vi "Diagnostics - Workspace Object.vi"() -> ()   [LabVIEW 2019, in "Diagnostics Workspace Object.lvlib"]
doc: "Sample numeric display item."
uses:
  Diagnostics Workspace Object.lvlib
  <vilib>/NI VeriStand/Display Template Support/DisplayTemplateSupport.llb/enum_Display Template Handler Minimal To Widget Msg.ctl
  <vilib>/NI VeriStand/Display Template Support/DisplayTemplateSupport.llb/enum_Display Template Handler Minimal To Workspace.ctl
  Workspace Shared/Types/Workspace.State.ctl
  Workspace Shared/Diagnostics Workspace Shared.lvlib
  <vilib>/NI VeriStand/Execution/Workspace/SystemStateRegEventRef.ctl
  <vilib>/NI VeriStand/Execution/Workspace/NI_VS Workspace ExecutionAPI.lvlib
  <vilib>/NI VeriStand/Execution/Workspace/WorkspaceAPI.ctl
  <vilib>/NI VeriStand/Execution/Workspace/SystemStateEventRef.ctl
  Workspace Shared/Types/UI.Refs.ctl
  <vilib>/NI VeriStand/Execution/Workspace/Target State.ctl
  <vilib>/NI VeriStand/Execution/Workspace/Target State Info.ctl
  Workspace Shared/Types/Workspace.SavedState.ctl
  Addon/Addon Shared/Types/Protocol.ctl
  Addon/Addon Shared/Diagnostics Addon Shared.lvlib
  <vilib>/NI VeriStand/Display Template Support/DisplayTemplateSupport.llb/sub_Display Template Handler Custom.vi
  NationalInstruments.VeriStand.ClientAPI
  NationalInstruments.VeriStand.SystemStorage
  Addon/Addon Shared/Types/Command.New.ctl
  APIs/Host Automation API/Diagnostics Host Automation API.lvlib
  Addon/Addon Shared/Types/DTC.Descriptor.Override.ctl
  Addon/Addon Shared/Types/Command.ReadDTC.ctl
  <vilib>/NI VeriStand/Execution/Workspace/NI VeriStand - Set Single Channel Value.vi
  <vilib>/NI VeriStand/Execution/Workspace/NI VeriStand - Get Multiple Channel Values.vi
  <vilib>/xnet/xnet.llb/XNET Frame Type CAN.ctl
  <vilib>/xnet/xnet.llb/XNET Frame CAN.ctl
  SubModules/CAN-Streaming-Support/UIs/Workspace Shared/Types/Host Stream Queue Command.ctl
  SubModules/CAN-Streaming-Support/UIs/Workspace Shared/CAN Stream Support Workspace Shared.lvlib
  SubModules/CAN-Streaming-Support/UIs/Workspace Shared/Types/Host Stream Queue Type.ctl
  SubModules/CAN-Streaming-Support/UIs/Workspace Shared/Types/Host Stream Queue Refs.ctl
  <vilib>/NI VeriStand/Display Template Support/DisplayTemplateSupport.llb/cluster_Screen Item Settings.ctl
  <vilib>/NI VeriStand/Display Template Support/DisplayTemplateSupport.llb/cluster_Graph Scale Settings.ctl
  <vilib>/NI VeriStand/Display Template Support/DisplayTemplateSupport.llb/cluster_Graph Plot Settings.ctl
panel:
  in  "Tab Control":enum32{"Cmd", "Raw", "Read DTCs"}(tab)
  out "Time Stamp":timestamp
  out "CAN Connected?":bool
  in  "Send":bool
  out "VeriStand Error":i64 format="%.0x"
  out "Success?":bool
  in  "Cmd":T1
  in  "Clear":bool
  out "Raw VeriStand Error":errorcluster
  out "Raw Error Byte":u8 format="%.0x"
  in  "Response Required?":bool
  in  "Send Raw":bool
  out "Raw Resp":u8[](array[numeric]) format="%.0x"
  in  "Raw Cmd":u8[](array[numeric]) format="%.0x"
  in  "DTC":u32
  in  "Status":u32
  in  "Failure":u32
  in  "Override Byte Lengths":bool
  in  "Extension":u32 format="%.0x"
  in  "Mask":u32 format="%.0x"
  in  "Mode":u32 format="%.0x"
  in  "Hex":bool=TRUE
  in  "DTCs":string(tree)
  in  "Read DTCs":bool
  out "Device":string
  in  "NIVS.System Definition Root":refnum<k24>
  in  "NIVS.Gateway IP Address":string
  in  "Item.Data":T2
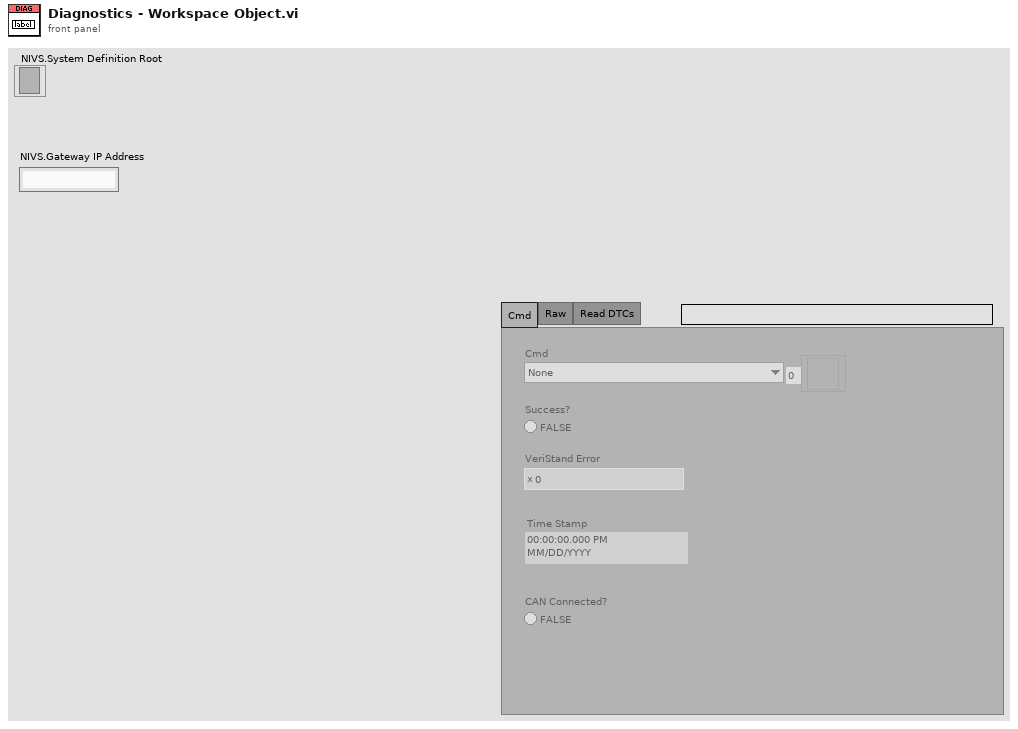
[diagram p1: front panel]
types:
  T1 = typedef "Diagnostics Addon Shared.lvlib/Command.New.ctl" = enum8{"None", "Clear Status Channels", "Read All DIDs", "Read All PIDs", "Configure and Start DPIDs", "Stop DPIDs"}
  T2 = typedef "cluster_Screen Item Settings.ctl" = cluster{"Template VI":string, "Position X":i32, "Position Y":i32, "Custom":string, "Show Title Bar":bool, "ID":i32, "Always On Top":bool, "Allow Resize":bool, "Allow Minimize":bool, "Allow Close":bool, "Size to Screen":bool, "Screen.ID":i32, "State":enum16{"Normal", "New"}, "Title":string, "Window Bounds":cluster{"[0]":i16, "[1]":i16, "[2]":i16, "[3]":i16}, "Channel Ref":u64, "Unit":string, "Default Units?":bool, "Flash Limit?":bool, "Color 1":u32, "Color 2":u32, "Color 3":u32, "Color 4":u32, "Bck Color":u32, "Fore Color":u32, "Limit 1":dbl, "Limit 2":dbl, "Limit 3":dbl, "Limit 4":dbl, "Limit Mode 1":i32, "Limit Mode 2":i32, "Limit Mode 3":i32, "Limit Mode 4":i32, "Scale Precision":i32, "Scale Min":dbl, "Scale Max":dbl, "Format":i32, "Precision":i32, "Background Type":i32, "IDs":i32[], "Units":string[], "Labels":string[], "Scale Factor":dbl, "Scale Offset":dbl, "YScale Index":u32[], "XScale":T3, "YScales":T3[], "Plots":T4[], "Update Period":dbl, "History Length":dbl, "My.Ref":refnum<vi>, "Is Control?":bool, "Channel Paths":string[], "Custom Data":variant}
  T3 = typedef "cluster_Graph Scale Settings.ctl" = cluster{"Format":u8, "Precision":u8, "Fit":u8, "Label":string, "Use Default Label":bool, "Label Visible":bool, "Min":dbl, "Max":dbl}
  T4 = typedef "cluster_Graph Plot Settings.ctl" = cluster{"Bar Style":u8, "Fill To":i16, "Fill/PtColor":u32, "Line Style":u8, "Line Width":u8, "Color":u32, "Interp":u8, "Point Style":u8}
  T5 = typedef "Diagnostics Workspace Shared.lvlib/Workspace.State.ctl" = cluster{"UI.Refs":T6, "Data.PreviousValues":dbl[], "Data.Read":string[], "CachedData.UserEvent":refnum<user-event>, "CachedData":T7, "Addon.Connected?":bool, "NIVS.SysDef":path, "NIVS.SysDefRoot":refnum<k24>, "NIVS.Workspace":T8, "NIVS.UserEventRefs":cluster{"Event Registration Refnum":refnum<event-registration>, "SystemChangeEventRef":T9, "NIVS.Workspace Event":refnum<event-registration>}, "NIVS.SystemStateRefs":T10, "NIVS.LaunchRef":refnum<user-event>, "Data.PendingChange?":bool, "Command.Channel":string, "Diagnostic Protocol":T11, "Channels.Found":bool, "Command.Connect":string, "Mode.Tool?":bool, "Stream.Qs":T12}
  T6 = typedef "Diagnostics Workspace Shared.lvlib/UI.Refs.ctl" = cluster{"Cmd":refnum<vi>, "Success?":refnum<vi>, "VeriStandError":refnum<vi>, "CAN Connected?":refnum<vi>, "DTC":refnum<vi>, "Status":refnum<vi>, "Failure":refnum<vi>, "Override Byte Lengths":refnum<vi>, "Response Required?":refnum<vi>, "Send":refnum<vi>, "Clear":refnum<vi>, "Send Raw":refnum<vi>, "Read DTCs":refnum<vi>, "Raw Cmd":refnum<vi>, "Extension":refnum<vi>, "Mode":refnum<vi>, "Mask":refnum<vi>, "Hex":refnum<vi>, "Raw Resp":refnum<vi>, "Raw Error Byte":refnum<vi>, "Raw VeriStand Error":refnum<vi>, "DTCs":refnum<vi>, "Time Stamp":refnum<vi>, "Device":refnum<vi>, "Pause":refnum<vi>, "Table Control":refnum<vi>, "Sort By ID":refnum<vi>, "Streaming Connected":refnum<vi>, "Enable Stream":refnum<vi>, "CAN State":refnum<vi>, "Direction Filter":refnum<vi>, "Type Filter":refnum<vi>, "Clear History":refnum<vi>, "Filter IDs":refnum<vi>, "Filter Location":refnum<vi>, "Reset Filter":refnum<vi>, "Log":refnum<vi>}
  T7 = typedef "Diagnostics Workspace Shared.lvlib/Workspace.SavedState.ctl" = cluster{"CD Path":string, "CD IP":string}
  T8 = typedef "NI_VS Workspace ExecutionAPI.lvlib/WorkspaceAPI.ctl" = refnum<k24>
  T9 = typedef "NI_VS Workspace ExecutionAPI.lvlib/SystemStateRegEventRef.ctl" = refnum<event-registration>
  T10 = typedef "NI_VS Workspace ExecutionAPI.lvlib/SystemStateEventRef.ctl" = cluster{"CustDatRef":refnum<user-event>, "EvtRef":refnum<k27>, "Target State User Event":refnum<user-event>}
  T11 = typedef "Diagnostics Addon Shared.lvlib/Protocol.ctl" = enum16{"GMLAN", "KWP-2000", "UDS", "User-Defined"}
  T12 = typedef "CAN Stream Support Workspace Shared.lvlib/Host Stream Queue Refs.ctl" = cluster{"Cmd Q":refnum<queue>, "XNET Frames":refnum<queue>}
  T13 = typedef "enum_Display Template Handler Minimal To Workspace.ctl" = cluster{"Operation":enum16{"SetCustomData", "DeleteItem"}, "Data":variant}
  T14 = typedef "enum_Display Template Handler Minimal To Widget Msg.ctl" = enum16{"Stop", "LaunchConfigDialog"}
  T15 = typedef "Diagnostics Addon Shared.lvlib/Command.ReadDTC.ctl" = cluster{"Extension":u32, "Mask":u32, "Mode/Status":u32, "Byte Lengths":T16}
  T16 = typedef "Diagnostics Addon Shared.lvlib/DTC.Descriptor.Override.ctl" = cluster{"Override":bool, "DTC":u32, "Status":u32, "Failure":u32}
  T17 = cluster{"Event Registration Refnum":refnum<event-registration>, "SystemChangeEventRef":T9, "NIVS.Workspace Event":refnum<event-registration>}
  T18 = typedef "Diagnostics Addon Shared.lvlib/UI.Refs.ctl" = cluster{"Cmd":refnum<vi>, "Success?":refnum<vi>, "VeriStandError":refnum<vi>, "CAN Connected?":refnum<vi>, "DTC":refnum<vi>, "Status":refnum<vi>, "Failure":refnum<vi>, "Override Byte Lengths":refnum<vi>, "Response Required?":refnum<vi>, "Send":refnum<vi>, "Clear":refnum<vi>, "Send Raw":refnum<vi>, "Read DTCs":refnum<vi>, "Raw Cmd":refnum<vi>, "Extension":refnum<vi>, "Mode":refnum<vi>, "Mask":refnum<vi>, "Hex":refnum<vi>, "Raw Resp":refnum<vi>, "Raw Error Byte":refnum<vi>, "Raw VeriStand Error":refnum<vi>, "DTCs":refnum<vi>, "Time Stamp":refnum<vi>, "Device":refnum<vi>, "Pause":refnum<vi>, "Table Control":refnum<vi>, "Sort By ID":refnum<vi>, "Streaming Connected":refnum<vi>, "Enable Stream":refnum<vi>, "CAN State":refnum<vi>, "Direction Filter":refnum<vi>, "Type Filter":refnum<vi>, "Clear History":refnum<vi>, "Filter IDs":refnum<vi>, "Filter Location":refnum<vi>, "Reset Filter":refnum<vi>, "Log":refnum<vi>}
  T19 = typedef "Diagnostics Addon Shared.lvlib/HostAutomation.Ref.ctl" = cluster{"TCP Comm":T20, "DTCs":T22}
  T20 = typedef "NI STM.lvlib/TCP Connection Info.ctl" = cluster{"connection ID":refnum<k5>, "meta data":T21[]}
  T21 = typedef "NI STM.lvlib/MetaDataElement.ctl" = string
  T22 = typedef "Diagnostics Addon Shared.lvlib/DTC.Codes.ctl" = cluster{"Value.Code":dbl[], "Value.String":string[], "Value.J2012String":string[], "Status.Code":dbl[], "Status.String":string[]}
  T23 = cluster{"resp":u8[], "error code":u8, "error out":errorcluster}
  T24 = typedef "Diagnostics Addon Shared.lvlib/Command.ReadDTC.DTCs.ctl" = cluster{"Timestamp":dbl, "DTC":dbl, "J2012 String":string, "DTC String":string, "Status":dbl, "Status String":string, "Add Data":dbl}
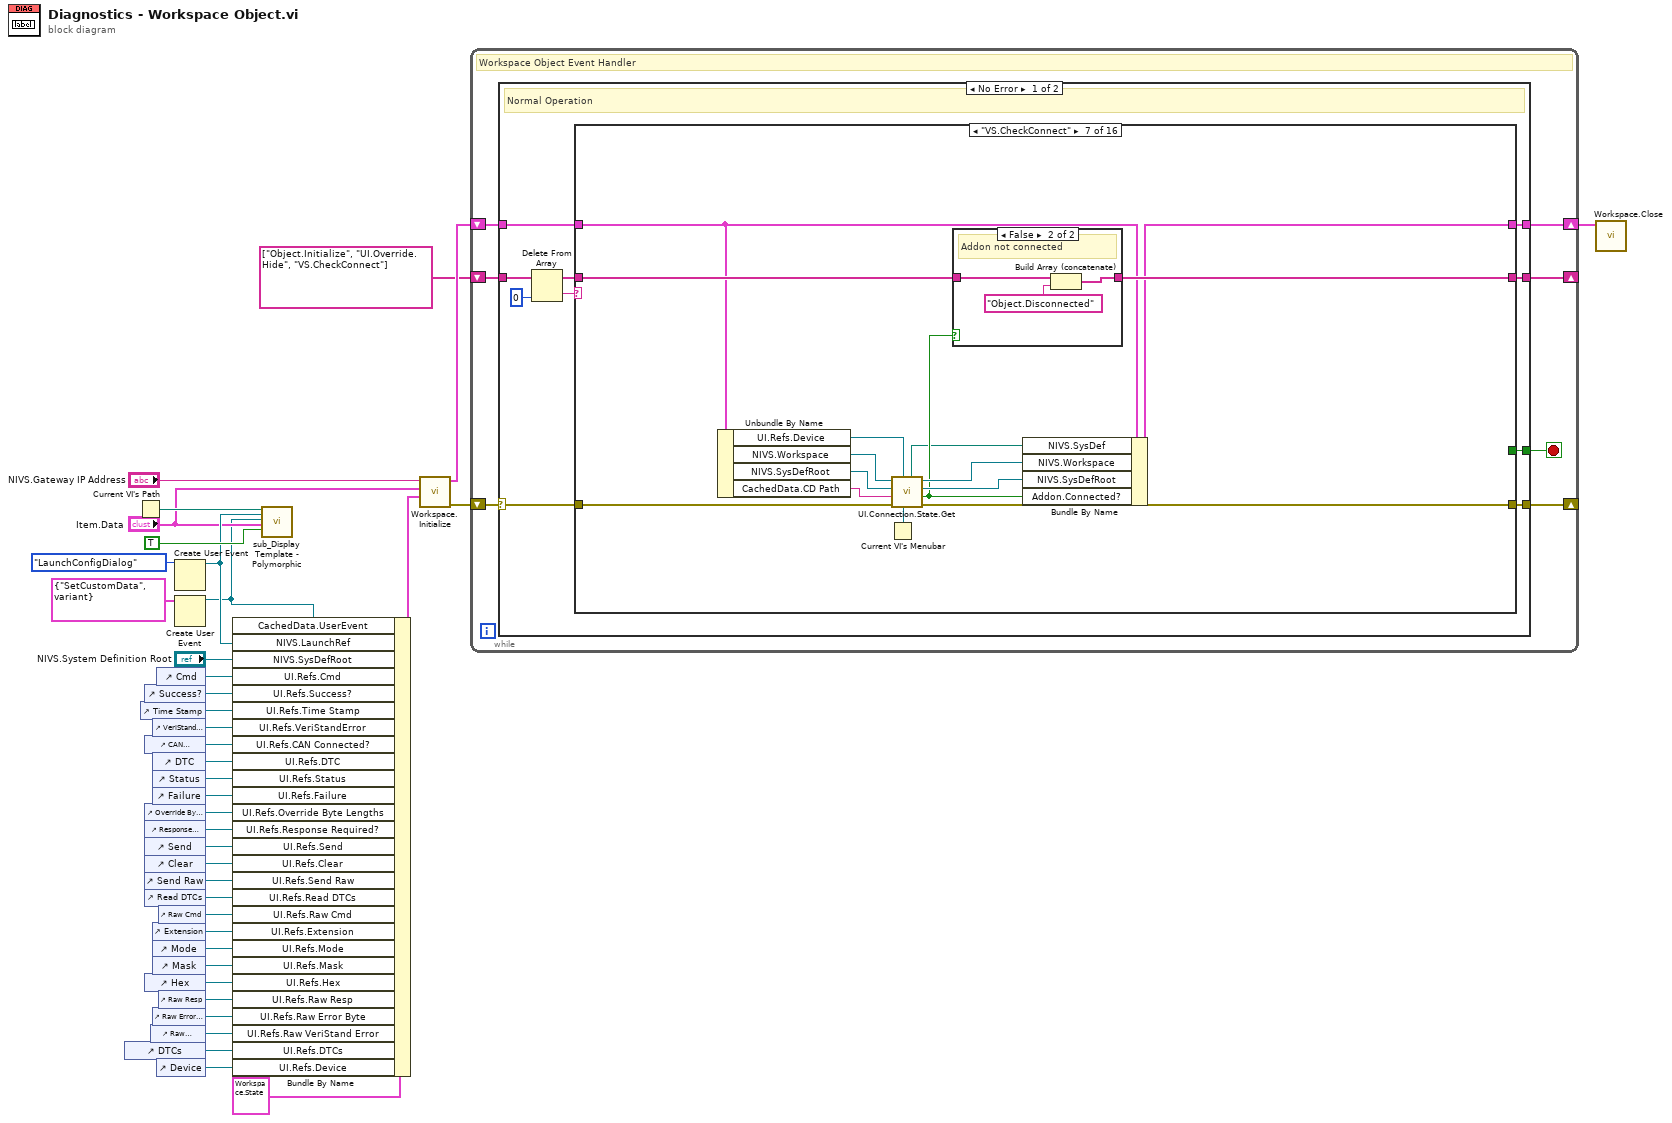
[diagram p0: block diagram]
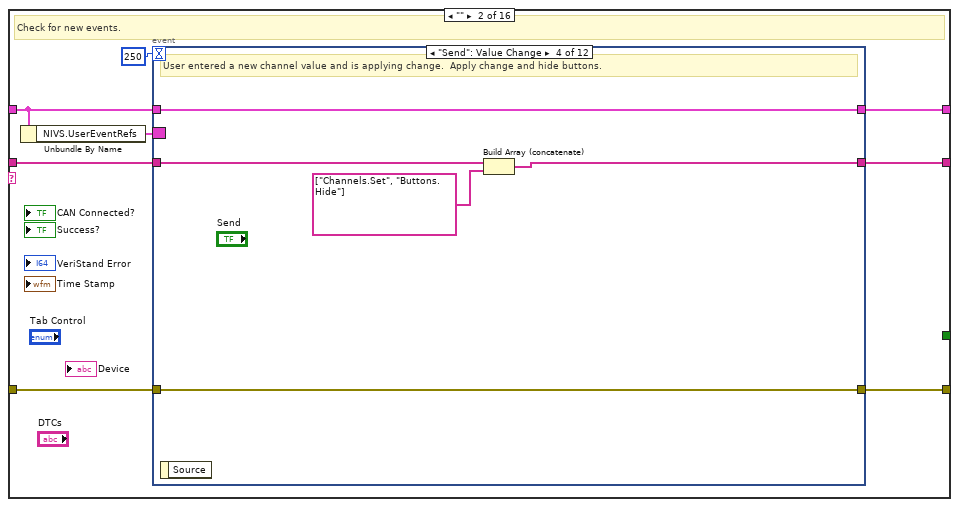
[diagram p3: hidden frame]
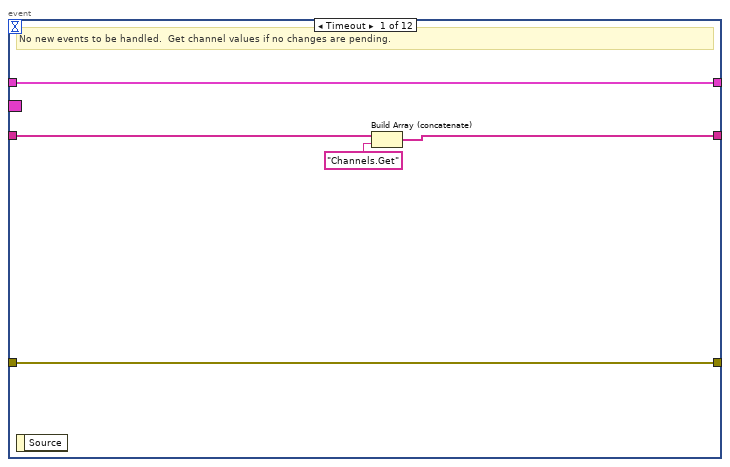
[diagram p4: hidden frame]
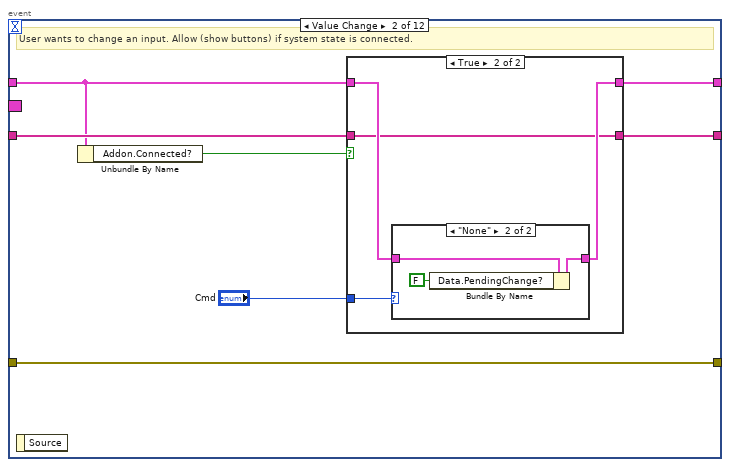
[diagram p5: hidden frame]
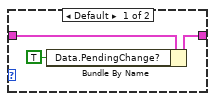
[diagram p7: hidden frame]
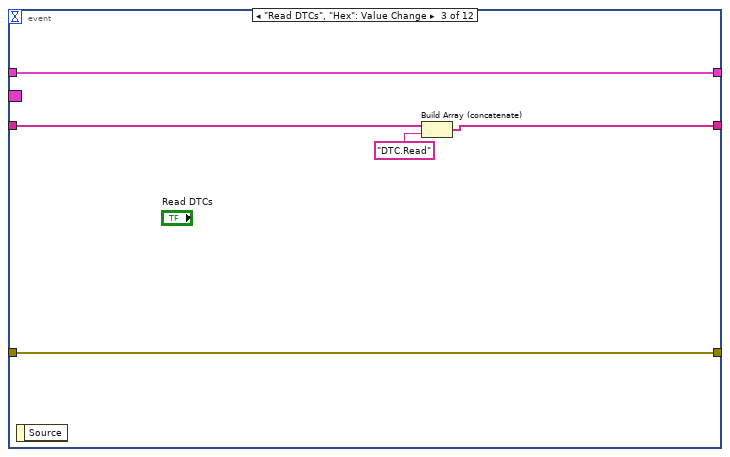
[diagram p8: hidden frame]
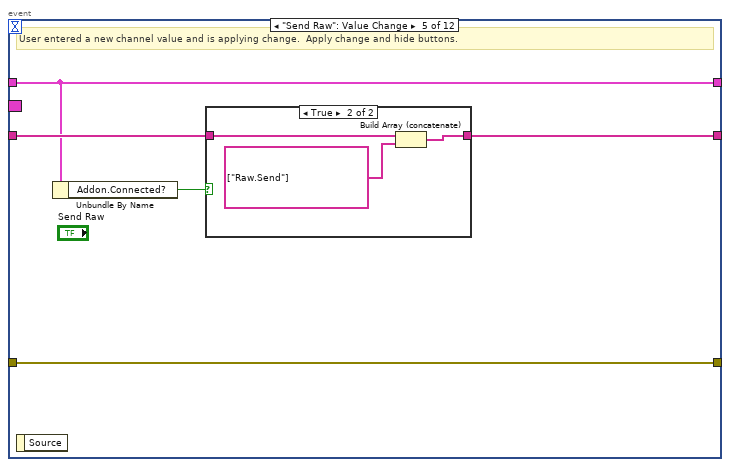
[diagram p9: hidden frame]
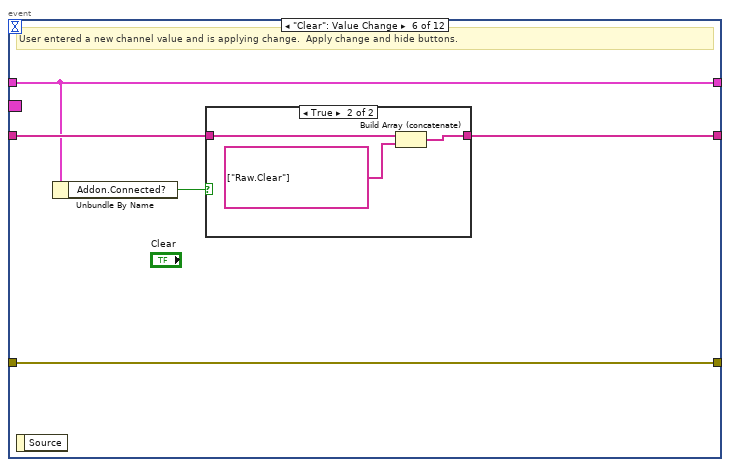
[diagram p11: hidden frame]
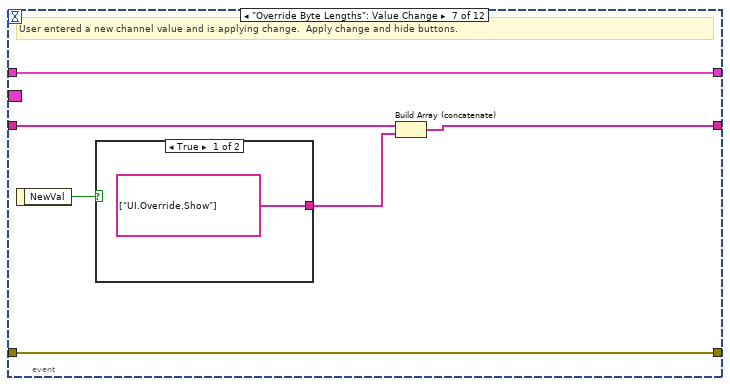
[diagram p13: hidden frame]
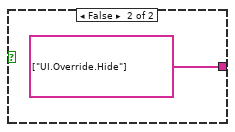
[diagram p14: hidden frame]
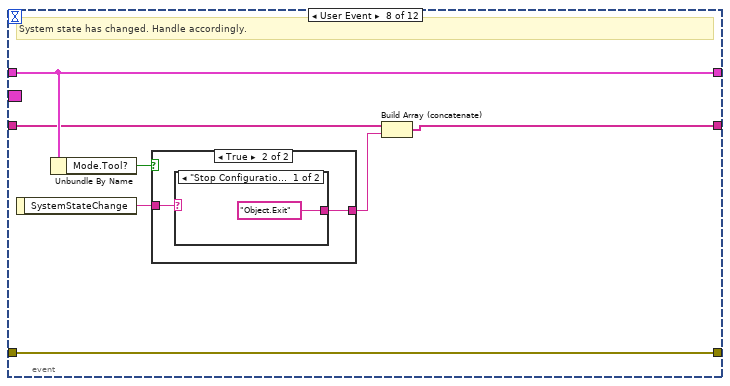
[diagram p15: hidden frame]
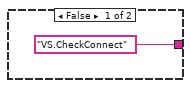
[diagram p16: hidden frame]
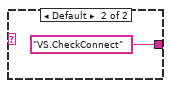
[diagram p17: hidden frame]
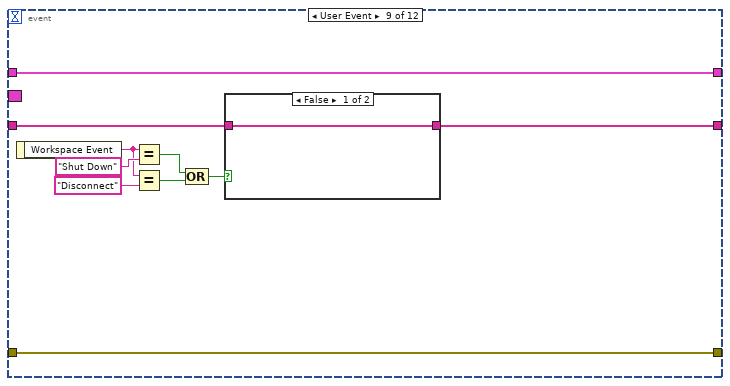
[diagram p18: hidden frame]
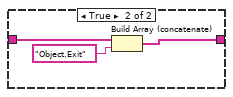
[diagram p19: hidden frame]
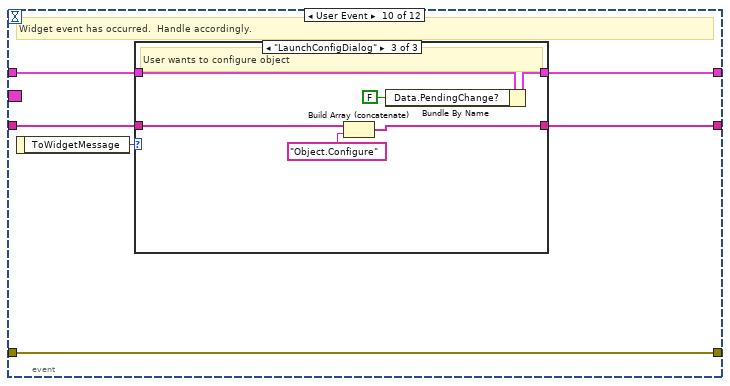
[diagram p20: hidden frame]
diagram:
  n1 = control-ref of="DTCs"() -> (w2:refnum<vi>)
  n2 = Current VI's Path() -> (path=w37:path)
  n3 = control-ref of="Time Stamp"() -> (w22:refnum<vi>)
  n4 = control-ref of="Success?"() -> (w23:refnum<vi>)
  n5 = control-ref of="CAN Connected?"() -> (w20:refnum<vi>)
  n6 = control-ref of="Override Byte Lengths"() -> (w16:refnum<vi>)
  n7 = control-ref of="Response Required?"() -> (w15:refnum<vi>)
  n8 = control-ref of="Send"() -> (w14:refnum<vi>)
  n9 = control-ref of="Clear"() -> (w13:refnum<vi>)
  n10 = control-ref of="Send Raw"() -> (w12:refnum<vi>)
  n11 = control-ref of="Read DTCs"() -> (w11:refnum<vi>)
  n12 = control-ref of="Hex"() -> (w6:refnum<vi>)
  n13 = control-ref of="Raw VeriStand Error"() -> (w3:refnum<vi>)
  n14 = control-ref of="VeriStand Error"() -> (w21:refnum<vi>)
  n15 = control-ref of="DTC"() -> (w19:refnum<vi>)
  n16 = control-ref of="Status"() -> (w18:refnum<vi>)
  n17 = control-ref of="Failure"() -> (w17:refnum<vi>)
  n18 = control-ref of="Extension"() -> (w9:refnum<vi>)
  n19 = control-ref of="Mode"() -> (w8:refnum<vi>)
  n20 = control-ref of="Mask"() -> (w7:refnum<vi>)
  n21 = control-ref of="Raw Error Byte"() -> (w4:refnum<vi>)
  n22 = control-ref of="Cmd"() -> (w24:refnum<vi>)
  n23 = control-ref of="Device"() -> (w1:refnum<vi>)
  n24 = control-ref of="Raw Cmd"() -> (w10:refnum<vi>)
  n25 = control-ref of="Raw Resp"() -> (w5:refnum<vi>)
  n26 = Create User Event(user event datatype=enum_Display_Template_Handler_Minimal_To_Widget_Msg."LaunchConfigDialog" ("ToWidgetMessage")) -> (user event=w34:refnum<user-event>)  [unwired: 1 in, 1 out]
  n27 = Create User Event(user event datatype=T13 {"Operation"=enum."SetCustomData", "Data"=variant} ("Data")) -> (user event=w30:refnum<user-event>)  [unwired: 1 in, 1 out]
  n28 = Bundle By Name(cluster=T5 {"UI.Refs"={"Cmd"=refnum, "Success?"=refnum, "VeriStandError"=refnum, "CAN Connected?"=refnum, "DTC"=refnum, "Status"=refnum, "Failure"=refnum, "Override Byte Lengths"=refnum, "Response Required?"=refnum, "Send"=refnum, "Clear"=refnum, "Send Raw"=refnum, "Read DTCs"=refnum, "Raw Cmd"=refnum, "Extension"=refnum, "Mode"=refnum, "Mask"=refnum, "Hex"=refnum, "Raw Resp"=refnum, "Raw Error Byte"=refnum, "Raw VeriStand Error"=refnum, "DTCs"=refnum, "Time Stamp"=refnum, "Device"=refnum, "Pause"=refnum, "Table Control"=refnum, "Sort By ID"=refnum, "Streaming Connected"=refnum, "Enable Stream"=refnum, "CAN State"=refnum, "Direction Filter"=refnum, "Type Filter"=refnum, "Clear History"=refnum, "Filter IDs"=refnum, "Filter Location"=refnum, "Reset Filter"=refnum, "Log"=refnum}, "Data.PreviousValues"=[], "Data.Read"=[], "CachedData.UserEvent"=refnum, "CachedData"={"CD Path"="", "CD IP"=""}, "Addon.Connected?"=FALSE, "NIVS.SysDef"=path "", "NIVS.SysDefRoot"=refnum, "NIVS.Workspace"=refnum, "NIVS.UserEventRefs"={"Event Registration Refnum"=refnum, "SystemChangeEventRef"=refnum, "NIVS.Workspace Event"=refnum}, "NIVS.SystemStateRefs"={"CustDatRef"=refnum, "EvtRef"=refnum, "Target State User Event"=refnum}, "NIVS.LaunchRef"=refnum, "Data.PendingChange?"=FALSE, "Command.Channel"="", "Diagnostic Protocol"=enum."GMLAN", "Channels.Found"=FALSE, "Command.Connect"="", "Mode.Tool?"=FALSE, "Stream.Qs"={"Cmd Q"=refnum, "XNET Frames"=refnum}}, "CachedData.UserEvent"=w30, "NIVS.LaunchRef"=w34, "NIVS.SysDefRoot"="NIVS.System Definition Root", "UI.Refs.Cmd"=w24, "UI.Refs.Success?"=w23, "UI.Refs.Time Stamp"=w22, "UI.Refs.VeriStandError"=w21, "UI.Refs.CAN Connected?"=w20, "UI.Refs.DTC"=w19, "UI.Refs.Status"=w18, "UI.Refs.Failure"=w17, "UI.Refs.Override Byte Lengths"=w16, "UI.Refs.Response Required?"=w15, "UI.Refs.Send"=w14, "UI.Refs.Clear"=w13, "UI.Refs.Send Raw"=w12, "UI.Refs.Read DTCs"=w11, "UI.Refs.Raw Cmd"=w10, "UI.Refs.Extension"=w9, "UI.Refs.Mode"=w8, "UI.Refs.Mask"=w7, "UI.Refs.Hex"=w6, "UI.Refs.Raw Resp"=w5, "UI.Refs.Raw Error Byte"=w4, "UI.Refs.Raw VeriStand Error"=w3, "UI.Refs.DTCs"=w2, "UI.Refs.Device"=w1) -> (w32:T5)
  n29 = call-poly <vilib>:"sub_Display Template - Polymorphic.vi"("Parent.Path"=w37, "ToWidgetEvent"=w34, "ToWorkspace"=w30, "Item.Data"="Item.Data", "Resizable"=TRUE) -> ()  [unwired: 1 in, 14 out]
  n30 = call "Workspace.Initialize.vi"("State Variables in"=w32, "Item.Data"="Item.Data", "NIVS.Gateway IP Address"="NIVS.Gateway IP Address") -> ("error out"=w29:errorcluster, "State Variables out"=w28:T5)  [unwired: 7 in]
  n31 = while {
    shift-right: [w44] -> _
    shift-left: string[] ["Object.Initialize", "UI.Override.Hide", "VS.CheckConnect"] -> [w45]
    shift-right: [w42] -> w27
    shift-left: w28 -> [w41]
    shift-right: [w43] -> _
    shift-left: w29 -> [w40]
    stop <- w46 stop-if-true
    # "Workspace Object Event Handler"
    n32 = case shown="No Error" w40 {
      selector: w40 -> [w47 w402]
      tunnel: [w56 _] -> w46
      tunnel: w45 -> [w54 w409]
      tunnel: [w51 w409] -> w44
      tunnel: [w50 w400] -> w43
      tunnel: [w49 w408] -> w42
      tunnel: w41 -> [w48 w408]
      frame No Error {
        # "Normal Operation"
        n33 = Delete From Array(array=w54, index=0) -> (deleted portion=w53:string, array with subset deleted=w52:string[])  [unwired: 1 in]
        n34 = case shown="\"VS.CheckConnect\"" w53 {
          tunnel: [_ _ _ _ _ _ _ TRUE _ _ _ _ _ _ _ _] -> w56
          tunnel: [w59 w66 w191 w196 w231 w248 w254 w273 w280 w293 w316 w334 w347 w370 w374 w399] -> w51
          tunnel: w47 -> [w58 w64 w184 w202 w227 w246 w259 w270 w279 w291 w315 w328 w341 w369 w373 w378]
          tunnel: w52 -> [w59 w65 w191 w195 w231 w248 w253 w273 w280 w293 w316 w334 w347 w370 w374 w399]
          tunnel: w48 -> [w57 w60 w188 w200 w232 w245 w251 w271 w276 w286 w313 w333 w346 w366 w372 w398]
          tunnel: [w58 w63 w187 w202 w216 w243 w258 w270 w279 w290 w314 w327 w340 w369 w373 w376] -> w50
          tunnel: [w57 w62 w188 w199 w214 w244 w252 w271 w276 w289 w312 w333 w346 w366 w372 w398] -> w49
          frame Default {
            # "Do nothing."
          }
          frame "" {
            # "Check for new events."
            n35 = Unbundle By Name(w60) -> ("NIVS.UserEventRefs"=w61:T17)
            n36 = event shown="[3] \"Send\": Value Change" {
              selector: w61 -> [_ _ _ _ _ _ _ _ _ _ _ _]
              dyn-events: _ -> [_ _ _ _ _ _ _ _ _ _ _ _]
              timeout: 250 -> [_ _ _ _ _ _ _ _ _ _ _ _]
              tunnel: [w70 w77 w92 w97 w104 w113 w123 w129 w142 w158 w172 w179] -> w66
              tunnel: w65 -> [w71 w78 w93 w98 w105 w114 w124 w131 w141 w157 w173 w180]
              tunnel: w64 -> [w72 w73 w96 w101 w106 w115 w125 w128 w149 w156 w176 w182]
              tunnel: [w72 w73 w96 w101 w106 w115 w125 w128 w149 w156 w176 w182] -> w63
              tunnel: [w69 w79 w95 w100 w103 w112 w122 w133 w148 w154 w175 w181] -> w62
              tunnel: w60 -> [w69 w76 w95 w100 w103 w112 w122 w133 w148 w155 w175 w181]
              event Timeout {
                # "No new events to be handled.  Get channel values if no changes are pending."
                n37 = event-data() -> ()  [unwired: 2 out]
                n38 = Build Array (concatenate)(w71, "Channels.Get") -> (w70:string[])
              }
              event Value Change {
                # "User wants to change an input. Allow (show buttons) if system state is connected."
                n39 = event-data() -> ()  [unwired: 2 out]
                n40 = Unbundle By Name(w76) -> ("Addon.Connected?"=w75:bool)
                n41 = case shown="True" w75 {
                  tunnel: w76 -> [w80 w85]
                  tunnel: [w80 w84] -> w79
                  tunnel: w78 -> [w81 w83]
                  tunnel: [w81 w83] -> w77
                  tunnel: "Cmd" -> [_ w82]
                  frame False {
                  }
                  frame True {
                    n42 = case shown="\"None\"" w82 {
                      tunnel: w85 -> [w87 w90]
                      tunnel: [w86 w89] -> w84
                      frame Default {
                        n43 = Bundle By Name(cluster=w87, "Data.PendingChange?"=TRUE ("Pending Change?")) -> (w86:T5)
                      }
                      frame "None" {
                        n44 = Bundle By Name(cluster=w90, "Data.PendingChange?"=FALSE ("Pending Change?")) -> (w89:T5)
                      }
                    }
                  }
                }
              }
              event "Read DTCs", "Hex": Value Change {
                n45 = event-data() -> ()  [unwired: 2 out]
                n46 = Build Array (concatenate)(w93, "DTC.Read") -> (w92:string[])
              }
              event "Send": Value Change {
                # "User entered a new channel value and is applying change.  Apply change and hide buttons."
                n47 = event-data() -> ()  [unwired: 2 out]
                n48 = Build Array (concatenate)(w98, string[] ["Channels.Set", "Buttons.Hide"]) -> (w97:string[])
              }
              event "Send Raw": Value Change {
                # "User entered a new channel value and is applying change.  Apply change and hide buttons."
                n49 = event-data() -> ()  [unwired: 2 out]
                n50 = Unbundle By Name(w103) -> ("Addon.Connected?"=w102:bool)
                n51 = case shown="True" w102 {
                  tunnel: w105 -> [w107 w109]
                  tunnel: [w107 w108] -> w104
                  frame False {
                  }
                  frame True {
                    n52 = Build Array (concatenate)(w109, string[] ["Raw.Send"]) -> (w108:string[])
                  }
                }
              }
              event "Clear": Value Change {
                # "User entered a new channel value and is applying change.  Apply change and hide buttons."
                n53 = event-data() -> ()  [unwired: 2 out]
                n54 = Unbundle By Name(w112) -> ("Addon.Connected?"=w111:bool)
                n55 = case shown="True" w111 {
                  tunnel: w114 -> [w116 w118]
                  tunnel: [w116 w117] -> w113
                  frame False {
                  }
                  frame True {
                    n56 = Build Array (concatenate)(w118, string[] ["Raw.Clear"]) -> (w117:string[])
                  }
                }
              }
              event "Override Byte Lengths": Value Change {
                # "User entered a new channel value and is applying change.  Apply change and hide buttons."
                n57 = event-data() -> ("NewVal"=w120:bool)  [unwired: 1 out]
                n58 = case shown="True" w120 {
                  tunnel: [string[] ["UI.Override.Show"] string[] ["UI.Override.Hide"]] -> w121
                  frame True {
                  }
                  frame False {
                  }
                }
                n59 = Build Array (concatenate)(w124, w121) -> (w123:string[])
              }
              event User Event {
                # "System state has changed. Handle accordingly."
                n60 = event-data() -> ("SystemStateChange"=w132:string)  [unwired: 1 out]
                n61 = Unbundle By Name(w133) -> ("Mode.Tool?"=w134:bool)
                n62 = case shown="True" w134 {
                  tunnel: ["VS.CheckConnect" w137] -> w130
                  tunnel: w132 -> [_ w136]
                  frame False {
                  }
                  frame True {
                    n63 = case shown="\"Stop Configuration\"" w136 {
                      tunnel: ["Object.Exit" "VS.CheckConnect"] -> w137
                      frame "Stop Configuration" {
                      }
                      frame Default {
                      }
                    }
                  }
                }
                n64 = Build Array (concatenate)(w131, w130) -> (w129:string[])
              }
              event User Event {
                n65 = event-data() -> ("Workspace Event"=w143:string)  [unwired: 1 out]
                n66 = Equal?(x=w143, y="Shut Down") -> (x = y?=w144:bool)
                n67 = Equal?(x=w143, y="Disconnect") -> (x = y?=w145:bool)
                n68 = Compound Arithmetic op=OR(w144, w145) -> (w140:bool)
                n69 = case shown="False" w140 {
                  tunnel: [w150 w152] -> w142
                  tunnel: w141 -> [w150 w151]
                  frame False {
                  }
                  frame True {
                    n70 = Build Array (concatenate)(w151, "Object.Exit") -> (w152:string[])
                  }
                }
              }
              event User Event {
                # "Widget event has occurred.  Handle accordingly."
                n71 = event-data() -> ("ToWidgetMessage"=w159:T14)  [unwired: 1 out]
                n72 = case shown="\"LaunchConfigDialog\"" w159 {
                  tunnel: [w161 w164 w170] -> w158
                  tunnel: w157 -> [w161 w165 w171]
                  tunnel: w155 -> [w160 w162 w168]
                  tunnel: [w160 w162 w167] -> w154
                  frame Default {
                    # "Do nothing."
                  }
                  frame "Stop" {
                    # "User exiting workspace or deleting object"
                    n73 = Build Array (concatenate)(w165, "Object.Exit") -> (w164:string[])
                  }
                  frame "LaunchConfigDialog" {
                    # "User wants to configure object"
                    n74 = Build Array (concatenate)(w171, "Object.Configure") -> (w170:string[])
                    n75 = Bundle By Name(cluster=w168, "Data.PendingChange?"=FALSE ("Pending Change?")) -> (w167:T5)
                  }
                }
              }
              event Menu Selection (User) {
                n76 = event-data() -> ("ItemTag"=w174:string)  [unwired: 1 out]
                n77 = Build Array (concatenate)(w173, w174) -> (w172:string[])
              }
              event Panel Close? {
                n78 = event-data() -> ()  [unwired: 5 out]
                n79 = Build Array (concatenate)(w180, "Object.Exit") -> (w179:string[])
                n80 = event-data("Discard?"=TRUE) -> ()  [unwired: 1 in, 1 out]
              }
            }
          }
          frame "Object.Initialize" {
            # "Initialize the workspace Object state variables and UI"
            n81 = Unbundle By Name(w188) -> ("UI.Refs.Override Byte Lengths"=w190:refnum<vi>, "UI.Refs.DTCs"=w186:refnum<vi>)
            n82 = local write "Tab Control"(0) -> ()
            n83 = invoke class="Tree (strict)" method="Edit Tree Items.Delete"(reference=w186, error in=w184, "Delete Children"=TRUE ("Delete Children?")) -> (error out=w185:errorcluster)  [unwired: 2 in, 4 out]
            n84 = property class="Bool (strict)"(reference=w190, error in=w185, "Value"=FALSE) -> (error out=w187:errorcluster)  [unwired: 1 out]
          }
          frame "Object.Configure" {
            # "Allow the user to select a control object to display"
            n85 = Unbundle By Name(w200) -> ("NIVS.SysDefRoot"=w194:refnum<k24>, "CachedData.CD Path"=w201:string)
            n86 = call "Workspace.Select.Dialog.vi"("CD Path"=w201, "NIVS.System Definition Root"=w194) -> ("Cancelled?"=w198:bool, "IP Address"=w193:string, "Custom Device Path Out"=w197:string)  [unwired: 7 in]
            n87 = case shown="True" w198 {
              tunnel: w200 -> [w209 w210]
              tunnel: [w208 w210] -> w199
              tunnel: w197 -> [w207 _]
              tunnel: [w205 w211] -> w196
              tunnel: w195 -> [w206 w211]
              tunnel: w193 -> [w203 _]
              frame False {
                # "Queue up required states and cache new controller path"
                n88 = Bundle By Name(cluster=w209, "CachedData.CD Path"=w207, "CachedData.CD IP"=w203) -> (w208:T5)
                n89 = Build Array (concatenate)(w206, string[] ["Cache.Update", "Object.Initialize", "UI.Override.Hide", "VS.CheckConnect"]) -> (w205:string[])
              }
              frame True {
                # "User canceled"
              }
            }
          }
          frame "Object.Connected" {
            # "System state is Connected. Get path to required channels and start UDP acquisition if channels found."
            n90 = Unbundle By Name(w232) -> ("CachedData.CD Path"=w213:string, "NIVS.SysDefRoot"=w226:refnum<k24>, "UI.Refs.Cmd"=w224:refnum<vi>)
            n91 = call "UI.Addon.Path.Parse.vi"("Cached Addon Path"=w213) -> ("Addon Path"=w212:string)  [unwired: 6 in, 4 out]
            n92 = call "Workspace.Channels.Create.vi"("CD Path"=w213) -> ("Read Channels"=w230:string[], "Command Channel"=w229:string)  [unwired: 9 in]
            n93 = call "Workspace.CAN.Protocol.Get.vi"("error in (no error)"=w227, "Path"=w212, "NIVS.SysDef Ref"=w226) -> ("error out"=w228:errorcluster, "Diagnostic Protocol"=w225:T11)  [unwired: 7 in]
            n94 = case shown="\"KWP-2000\", \"UDS\"" w225 {
              tunnel: [w238 w240 w242] -> w223
              tunnel: [bool[] [TRUE, TRUE, TRUE] bool[] [TRUE, TRUE, TRUE] bool[] [TRUE, TRUE, FALSE]] -> w220
              frame "GMLAN" {
                w238 = T1[] [] items=["None", "Clear Status Channels", "Read All DIDs", "Read All PIDs", "Configure and Start DPIDs", "Stop DPIDs"] ("Disabled Items []")
              }
              frame "KWP-2000", "UDS" {
                w240 = T1[] [enum."Read All PIDs", enum."Configure and Start DPIDs", enum."Stop DPIDs"] items=["None", "Clear Status Channels", "Read All DIDs", "Read All PIDs", "Configure and Start DPIDs", "Stop DPIDs"] ("Disabled Items []")
              }
              frame "User-Defined" {
                w242 = T1[] [enum."Read All DIDs", enum."Read All PIDs", enum."Configure and Start DPIDs", enum."Stop DPIDs"] items=["None", "Clear Status Channels", "Read All DIDs", "Read All PIDs", "Configure and Start DPIDs", "Stop DPIDs"] ("Disabled Items []")
              }
            }
            n95 = Bundle By Name(cluster=w232, "Command.Channel"=w229, "Data.Read"=w230, "Diagnostic Protocol"=w225) -> (w215:T5)
            n96 = property class="Enum (strict)"(reference=w224, error in=w228, "Disabled Items []"=w223) -> (error out=w222:errorcluster)  [unwired: 1 out]
            n97 = property on="Tab Control" class="TabCtl (strict)"(error in=w222) -> (error out=w219:errorcluster, "Pages"=w221:refnum<vi>[])  [unwired: 1 in, 1 out]
            n98 = for {
              tunnel: w221 -> [w236] mode=indexing
              tunnel: w220 -> [w235] mode=indexing
              shift-right: [w233] -> w217
              shift-left: w219 -> [w234]
              n99 = property class="Page"(reference=w236, error in=w234, "PageVis"=w235) -> (error out=w233:errorcluster)  [unwired: 1 out]
            }
            n100 = call "Workspace.UI.DisableState.Set.vi"("Enable?"=TRUE, "error in (no error)"=w217, "State Variables in"=w215) -> ("error out"=w216:errorcluster, "State Variables out"=w214:T5)  [unwired: 7 in]
          }
          frame "Object.Disconnected" {
            n101 = call "Workspace.UI.DisableState.Set.vi"("Enable?"=FALSE, "error in (no error)"=w246, "State Variables in"=w245) -> ("error out"=w243:errorcluster, "State Variables out"=w244:T5)  [unwired: 7 in]
          }
          frame "VS.CheckConnect" {
            n102 = Unbundle By Name(w251) -> ("UI.Refs.Device"=w250:refnum<vi>, "NIVS.Workspace"=w262:T8, "NIVS.SysDefRoot"=w261:refnum<k24>, "CachedData.CD Path"=w260:string)
            n103 = Current VI's Menubar() -> (w263:refnum<k9>)
            n104 = call "UI.Connection.State.Get.vi"("Menu Ref"=w263, "Name Ref"=w250, "error in (no error)"=w259, "Addon Path in"=w260, "NIVS.System Definition Root in"=w261, "NIVS.Workspace Ref in"=w262) -> ("error out"=w258:errorcluster, "Addon Connected?"=w255:bool, "NIVS.System Definition Root out"=w256:refnum<k24>, "NIVS.Workspace Ref out"=w257:T8, "System Definition File"=w249:path)  [unwired: 1 in]
            n105 = case shown="False" w255 {
              tunnel: [w266 w269] -> w254
              tunnel: w253 -> [w264 w267]
              frame True {
                # "Addon connected"
                n106 = Build Array (concatenate)(w264, "Object.Connected") -> (w266:string[])
              }
              frame False {
                # "Addon not connected"
                n107 = Build Array (concatenate)(w267, "Object.Disconnected") -> (w269:string[])
              }
            }
            n108 = Bundle By Name(cluster=w251, "NIVS.SysDef"=w249, "NIVS.Workspace"=w257, "NIVS.SysDefRoot"=w256, "Addon.Connected?"=w255) -> (w252:T5)
          }
          frame "Object.Exit" {
            # "Stop current loop.  Queue Stop Acq and Exit to UDP loop."
          }
          frame "Cache.Update" {
            # "Cache any data needing to be permenantly stored with the workspace object."
            n109 = Unbundle By Name(w276) -> ("CachedData.UserEvent"=w274:refnum<user-event>, "CachedData"=w275:T7)
            n110 = Bundle By Name(cluster=T13 {"Operation"=enum."SetCustomData", "Data"=variant} ("event data"), "Data"=w275) -> (w277:T13)
            n111 = Generate User Event(user event=w274, event data cluster=w277) -> ()  [unwired: 2 in, 2 out]
          }
          frame "Channels.Get" {
            # "Get the current slow speed channel values from VeriStand if no pending change, data paths are valid and system state is connected."
            n112 = Unbundle By Name(w286) -> ("UI.Refs"=w281:T18, "Data.PendingChange?"=w282:bool, "Addon.Connected?"=w292:bool, "NIVS.Workspace"=w288:T8, "Data.Read"=w287:string[])
            n113 = case shown="False" w292 {
              tunnel: w291 -> [w299 w305]
              tunnel: [w299 w304] -> w283
              tunnel: w288 -> [w298 w303]
              tunnel: [w298 w302] -> w285
              tunnel: w287 -> [w297 w301]
              tunnel: [w294 w300] -> w284
              frame False {
                # "Do Nothing."
                n114 = Array Size(array=w297) -> (size(s)=w296:i32)
                n115 = Initialize Array(0.0 ("element"), w296) -> (w294:dbl[])
              }
              frame True {
                # "Connected & paths valid"
                n116 = call-poly <vilib>:"NI VeriStand - Get Channel Value.vi"("error in (no error)"=w305, "Channels"=w301, "WorkspaceManager in"=w303) -> ("error out"=w304:errorcluster, "Values"=w300:dbl[], "WorkspaceManager out"=w302:T8)  [unwired: 6 in]
              }
            }
            n117 = call "Workspace.UI.Update.vi"("error in (no error)"=w283, "Data.PendingChange?"=w282, "Values"=w284, "UI.Refs"=w281) -> ("error out"=w290:errorcluster)  [unwired: 7 in]
            n118 = Bundle By Name(cluster=w286, "NIVS.Workspace"=w285, "Data.PreviousValues"=w284) -> (w289:T5)
          }
          frame "Channels.Set" {
            # "Set Channels if data paths are valid and system state is connected and there is a change in the data value."
            n119 = Unbundle By Name(w313) -> ("Addon.Connected?"=w309:bool, "NIVS.Workspace"=w308:T8, "Command.Channel"=w306:string, "UI.Refs"=w307:T18)
            n120 = case shown="True" w309 {
              tunnel: w315 -> [w318 w320]
              tunnel: [w318 w326] -> w314
              tunnel: w308 -> [w317 w325]
              tunnel: [w317 w324] -> w310
              tunnel: w306 -> [_ w323]
              tunnel: w307 -> [_ w321]
              frame False {
                # "Do nothing"
              }
              frame True {
                # "Connected & paths valid"
                n121 = call "Workspace.UI.Pull.vi"("error in (no error)"=w320, "UI.Refs"=w321) -> ("error out"=w319:errorcluster, "Value"=w322:dbl)  [unwired: 8 in]
                n122 = call-poly <vilib>:"NI VeriStand - Set Channel Value.vi"("error in (no error)"=w319, "Value"=w322, "Channel"=w323, "WorkspaceManager in"=w325) -> ("error out"=w326:errorcluster, "WorkspaceManager out"=w324:T8)  [unwired: 6 in]
              }
            }
            n123 = Bundle By Name(cluster=w313, "Data.PendingChange?"=FALSE ("Pending Change?"), "NIVS.Workspace"=w310) -> (w312:T5)
          }
          frame "UI.Override.Hide" {
            # "Reset slow speed channel displayed values."
            n124 = Unbundle By Name(w333) -> ("UI.Refs.DTC"=w332:refnum<vi>, "UI.Refs.Status"=w331:refnum<vi>, "UI.Refs.Failure"=w330:refnum<vi>)
            n125 = Build Array(w332, w331, w330) -> (w329:refnum<vi>[])
            n126 = for {
              tunnel: w329 -> [w339] mode=indexing
              shift-right: [w337] -> w327
              shift-left: w328 -> [w338]
              n127 = property class="DigNum (strict)"(reference=w339, error in=w338, "Visible"=FALSE, "Value"=u32 0) -> (error out=w337:errorcluster)  [unwired: 1 out]
            }
          }
          frame "UI.Override.Show" {
            # "Reset slow speed channel displayed values."
            n128 = Unbundle By Name(w346) -> ("UI.Refs.DTC"=w345:refnum<vi>, "UI.Refs.Status"=w344:refnum<vi>, "UI.Refs.Failure"=w343:refnum<vi>)
            n129 = Build Array(w345, w344, w343) -> (w342:refnum<vi>[])
            n130 = for {
              tunnel: w342 -> [w351] mode=indexing
              shift-right: [w349] -> w340
              shift-left: w341 -> [w350]
              n131 = property class="DigNum (strict)"(reference=w351, error in=w350, "Visible"=TRUE) -> (error out=w349:errorcluster)  [unwired: 1 out]
            }
          }
          frame "Raw.Send" {
            # "Reset slow speed channel displayed values."
            n132 = Unbundle By Name(w366) -> ("CachedData.CD IP"=w355:string, "CachedData.CD Path"=w353:string)
            n133 = call "UI.Addon.Path.Parse.vi"("Cached Addon Path"=w353) -> ("Addon Name"=w352:string)  [unwired: 6 in, 4 out]
            n134 = Bundle By Name(cluster=cluster{"cmd":u8[], "require response?":bool} {"cmd"=[], "require response?"=TRUE} ("Cmd"), "cmd"="Raw Cmd", "require response?"="Response Required?") -> (w364:cluster{"cmd":u8[], "require response?":bool})
            n135 = call "Connect.vi"("Addon Name"=w352, "Address"=w355) -> ("error out"=w361:errorcluster, "Ref"=w367:T19)  [unwired: 8 in]
            n136 = call "PassThru.vi"("error in (no error)"=w361, "timeout ms (1000)"=2500, "Cmd"=w364, "Ref"=w367) -> ("error out"=w360:errorcluster, "Resp"=w359:T23, "Ref"=w368:T19)  [unwired: 5 in]
            n137 = Unbundle By Name(w359) -> ("resp"=→"Raw Resp":u8[], "error code"=→"Raw Error Byte":u8, "error out"=→"Raw VeriStand Error":errorcluster)
            n138 = call "Disconnect.vi"("error in"=w360, "Ref"=w368) -> ()  [unwired: 9 in, 1 out]
          }
          frame "Raw.Clear" {
            n139 = local write "Raw Cmd"(u8[] [] ("Cmd")) -> ()
          }
          frame "DTC.Read" {
            # "Reset slow speed channel displayed values."
            n140 = Unbundle By Name(w398) -> ("CachedData.CD IP"=w396:string, "CachedData.CD Path"=w397:string)
            n141 = Bundle By Name(cluster=T15 {"Extension"=0, "Mask"=0, "Mode/Status"=0, "Byte Lengths"={"Override"=FALSE, "DTC"=0, "Status"=0, "Failure"=0}} ("Options (KWP/UDS Only)"), "Extension"="Extension", "Mask"="Mask", "Mode/Status"="Mode", "Byte Lengths.Override"="Override Byte Lengths", "Byte Lengths.DTC"="DTC", "Byte Lengths.Status"="Status", "Byte Lengths.Failure"="Failure") -> (w390:T15)
            n142 = call "UI.Addon.Path.Parse.vi"("Cached Addon Path"=w397) -> ("Addon Name"=w375:string)  [unwired: 6 in, 4 out]
            n143 = call "Connect.vi"("Addon Name"=w375, "Address"=w396) -> ("error out"=w394:errorcluster, "Ref"=w395:T19)  [unwired: 8 in]
            n144 = call "ReadDTCs.vi"("error in (no error)"=w394, "timeout ms (1000)"=2500, "Options (KWP/UDS Only)"=w390, "Ref"=w395) -> ("error out"=w393:errorcluster, "Active DTCs"=w380:T24[], "Ref"=w392:T19)  [unwired: 5 in]
            n145 = call "Disconnect.vi"("error in"=w393, "Ref"=w392) -> ("error out"=w385:errorcluster)  [unwired: 9 in]
            n146 = control-ref of="DTCs"() -> (w377:refnum<vi>)
            n147 = call <vilib>:"Simple Error Handler.vi"("error in (no error)"=w385) -> ()  [unwired: 4 in, 5 out]
            n148 = call "Workspace.DTC.Update.vi"("Hex"="Hex", "error in"=w378, "Active DTCs"=w380, "DTCs"=w377) -> ("error out"=w376:errorcluster)  [unwired: 7 in]
          }
        }
      }
      frame Error {
        # "Handle Errors."
        n149 = Unbundle By Name(w402) -> ("code"=w406:i32)
        n150 = Equal?(x=-307654, y=w406) -> (x = y?=w404:bool)
        n151 = Select(t=errorcluster {"status"=FALSE, "code"=0, "source"=""}, s=w404, f=w402) -> (s? t:f=w401:errorcluster)
        n152 = call <vilib>:"Simple Error Handler.vi"("error in (no error)"=w401) -> ("error out"=w407:errorcluster)  [unwired: 4 in, 4 out]
        n153 = call <vilib>:"Clear Errors.vi"("error in (no error)"=w407) -> ("error out"=w400:errorcluster)  [unwired: 5 in, 1 out]
      }
    }
  }
  n154 = call "Workspace.Close.vi"("State Variables in"=w27) -> ()  [unwired: 11 in]
